vi "numeric_data.get.vi"(8 "error in (no error)":errorcluster, 11 "midi-file-event.meta in":refnum<class "midi-file-event.meta.lvclass">) -> (0 "error out":errorcluster, 2 "Numeric Data":i32[](array[numeric]), 3 "midi-file-event.meta out":refnum<class "midi-file-event.meta.lvclass">)   [LabVIEW 2020, in "midi-file-event.meta.lvclass"]
uses:
  midi-file-event.meta.lvclass
  midi-file-event.meta.lvclass/midi-file-event.meta.ctl
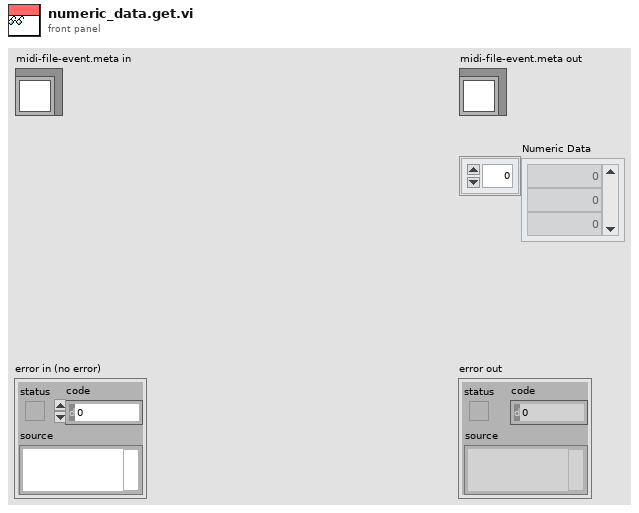
[diagram p1: front panel]
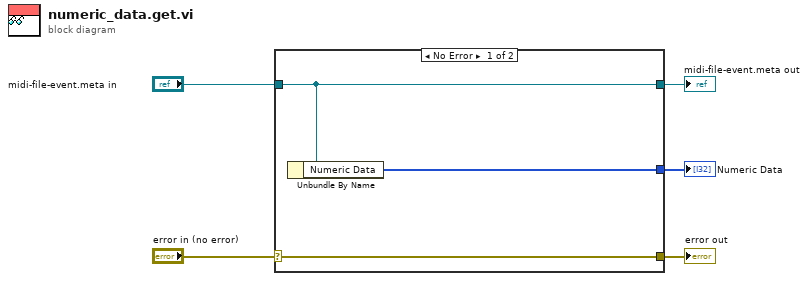
[diagram p0: block diagram]
diagram:
  n1 = case shown="No Error" "error in (no error)" {
    selector: "error in (no error)" -> [w8 w9]
    tunnel: [w8 w9] -> w4
    tunnel: [w7 w10] -> w2
    tunnel: "midi-file-event.meta in" -> [w7 w10]
    tunnel: [w6 _] -> w1
    frame No Error {
      n2 = Unbundle By Name(w7) -> ("Numeric Data"=w6:i32[])
    }
    frame Error {
    }
  }
  "error out" <- w4
  "midi-file-event.meta out" <- w2
  "Numeric Data" <- w1
